vi "Vision_Processing_R_R10.vi"(0 "Current State":T2(ring), 1 "Image Dst":T6=refnum, 2 "Inpute Image":T6=refnum, 3 "Startup Flag":bool, 5 "Current ROI Descriptor":T11={"Global Rectangle"=[0, 0, 640, 480], "Contours"=[{"ID"=enum."External", "Type"=12, "Coordinates"=[0, 0, 640, 480, 0]}]} {"Contours"."Type" items=["No Selection", "Point", "Line", "Rectangle", "Oval", "Polygon", "Freehand Region", "Annulus", "Unused2", "Unused3", "Broken Line", "Freehand Line", "Rotated Rectangle"]}, 6 "Avg Score - Last":dbl=923.3457641601562, 7 "error in (no error)":errorcluster, 8 "Current Settings":T9={"Curve Parameters"={"Extraction Mode"=1, "Edge Threshold"=150, "Edge Filter Size"=0, "Min Length"=15, "Row Search Step Size"=10, "Col Search Step Size"=10, "Max Endpoint Gap"=2, "Closed"=TRUE, "Subpixel"=TRUE}, "Match Mode"={"Rotation"=TRUE, "Scale"=TRUE, "Occlusion"=FALSE, "Reserved"=FALSE, "Reserved"=FALSE, "Reserved"=FALSE}, "Range Settings"=[{"Match Constraints"=0, "Min"=-5.0, "Max"=5.0}, {"Match Constraints"=1, "Min"=20.0, "Max"=170.0}, {"Match Constraints"=2, "Min"=0.0, "Max"=20.0}], "Number of Matches"=1, "Minimum Match Score"=800.0, "SubPixel Accuracy"=TRUE, "Adv. Geometric Match Options 2"=[{"Setup Data Item"=20, "Item Value"=0.0}, {"Setup Data Item"=22, "Item Value"=1.0}]} {"Curve Parameters"."Extraction Mode" items=["Normal", "Uniform Regions"]; "Curve Parameters"."Edge Filter Size" items=["Fine", "Normal", "Contour Tracing"]; "Curve Parameters"."Max Endpoint Gap" min=0; "Curve Parameters"."Col Search Step Size" min=1 max=255 step=1; "Curve Parameters"."Row Search Step Size" min=1 max=255 step=1; "Curve Parameters"."Min Length" min=0; "Curve Parameters"."Edge Threshold" min=1 max=350 step=1; "Range Settings"."Max" format="%.2f"; "Range Settings"."Min" format="%.2f"; "Range Settings"."Match Constraints" items=["Rotation Angle (degrees)", "Scale Factor (%)", "Occlusion (%)"]; "Adv. Geometric Match Options 2"."Setup Data Item" items=["Curve Extraction Mode", "Curve Edge Threshold", "Curve Edge Filter Size", "Min Curve Length", "Curve Row Search Step Size", "Curve Col Search Step Size", "Curve Max Endpoint Gap", "Extract Closed Curves", "Enable Subpixel Curve Extraction", "Enable Correlation Score", "Enable Subpixel Accuracy", "Subpixel Iterations", "Subpixel Tolerance", "Initial Match List Length", "Enable Target Template Curve Score", "Min Match Separation Distance", "Min Match Separation Angle", "Min Match Separation Scale", "Max Match Overlap", "Enable Coarse Result", "Enable Calibration Support", "Enable Contrast Reversal", "Search Strategy", "Refinement Match Factor", "Subpixel Match Factor"]}, 9 "Sub Beacon Search Enable":bool[](array[boolean])=[FALSE, FALSE, FALSE, FALSE, FALSE], 10 "History Data - IN":T5={"Valid Beacon History - in"=[FALSE, FALSE, TRUE, FALSE, FALSE, FALSE, FALSE, FALSE, FALSE, FALSE, FALSE, FALSE, FALSE, FALSE, FALSE, TRUE, FALSE, FALSE, FALSE, FALSE], "Valid Score History"=[0.0, 0.0, 934.5453491210938, 891.6079711914062, 0.0, 0.0, 0.0, 0.0, 0.0, 0.0, 0.0, 0.0, 884.2328491210938, 0.0, 0.0, 902.6854858398438, 0.0, 0.0, 0.0, 0.0], "Valid Scale History"=[0.0, 0.0, 51.11858367919922, 10.0, 0.0, 0.0, 0.0, 0.0, 0.0, 0.0, 0.0, 0.0, 10.0, 0.0, 0.0, 55.87311935424805, 0.0, 0.0, 0.0, 0.0]} {"Valid Scale History" format="%#_13g"; "Valid Score History" format="%#_13g"}, 13 "Avg Scale - Last":dbl=54.029449462890625, 16 "History Size":i32=20) -> (11 "Avg Scale":dbl=54.029449462890625, 12 "Avg Score":dbl=923.3457641601562, 14 "Tracking Info 1":T1={"Tracking Coordinates"={"X"=0.0, "Y"=0.0}, "Current Valid"=FALSE, "Current State - Out"=enum."Sub - 2", "Setting Values"={"Min Scale"=17.429317474365234, "Max Scale"=90.62958145141602, "Min Score"=850.0}}, 15 "Next Main ROI Descriptor":T3={"Global Rectangle"=[0, 0, 640, 480], "Contours"=[{"ID"=enum."External", "Type"=12, "Coordinates"=[0, 0, 640, 480, 0]}]} {"Contours"."Type" items=["No Selection", "Point", "Line", "Rectangle", "Oval", "Polygon", "Freehand Region", "Annulus", "Unused2", "Unused3", "Broken Line", "Freehand Line", "Rotated Rectangle"]}, 17 "Beacon - Scales":sgl[](array[numeric]), 18 "History Data - Out":T4={"Valid Beacon History\nOut"=[FALSE, FALSE, TRUE, FALSE, FALSE, FALSE, FALSE, FALSE, FALSE, FALSE, FALSE, FALSE, FALSE, FALSE, FALSE, TRUE, FALSE, FALSE, FALSE, FALSE], "Valid Score History\nOut"=[0.0, 0.0, 934.5453491210938, 891.6079711914062, 0.0, 0.0, 0.0, 0.0, 0.0, 0.0, 0.0, 0.0, 884.2328491210938, 0.0, 0.0, 902.6854858398438, 0.0, 0.0, 0.0, 0.0], "Valid Scale History\nOut"=[0.0, 0.0, 51.11858367919922, 10.0, 0.0, 0.0, 0.0, 0.0, 0.0, 0.0, 0.0, 0.0, 10.0, 0.0, 0.0, 55.87311935424805, 0.0, 0.0, 0.0, 0.0]} {"Valid Scale History\nOut" format="%#_13g"; "Valid Score History\nOut" format="%#_13g"}, 19 "Y Coordinates":sgl[](array[numeric]), 20 "Beacons Found":bool[](array[boolean]), 21 "X Coordinates":sgl[](array[numeric]), 22 "Next State":T2(ring), 23 "Lock Status":bool, 24 "Startup Flag - out":bool, 25 "New Settings":T9={"Curve Parameters"={"Extraction Mode"=1, "Edge Threshold"=150, "Edge Filter Size"=0, "Min Length"=15, "Row Search Step Size"=10, "Col Search Step Size"=10, "Max Endpoint Gap"=2, "Closed"=TRUE, "Subpixel"=TRUE}, "Match Mode"={"Rotation"=TRUE, "Scale"=TRUE, "Occlusion"=FALSE, "Reserved"=FALSE, "Reserved"=FALSE, "Reserved"=FALSE}, "Range Settings"=[{"Match Constraints"=0, "Min"=-5.0, "Max"=5.0}, {"Match Constraints"=1, "Min"=20.0, "Max"=170.0}, {"Match Constraints"=2, "Min"=0.0, "Max"=20.0}], "Number of Matches"=1, "Minimum Match Score"=800.0, "SubPixel Accuracy"=TRUE, "Adv. Geometric Match Options 2"=[{"Setup Data Item"=20, "Item Value"=0.0}, {"Setup Data Item"=22, "Item Value"=1.0}]} {"Curve Parameters"."Extraction Mode" items=["Normal", "Uniform Regions"]; "Curve Parameters"."Edge Filter Size" items=["Fine", "Normal", "Contour Tracing"]; "Curve Parameters"."Max Endpoint Gap" min=0; "Curve Parameters"."Col Search Step Size" min=1 max=255 step=1; "Curve Parameters"."Row Search Step Size" min=1 max=255 step=1; "Curve Parameters"."Min Length" min=0; "Curve Parameters"."Edge Threshold" min=1 max=350 step=1; "Range Settings"."Max" format="%.2f"; "Range Settings"."Min" format="%.2f"; "Range Settings"."Match Constraints" items=["Rotation Angle (degrees)", "Scale Factor (%)", "Occlusion (%)"]}, 27 "Right Image 2":T6(plugin-control))   [LabVIEW 2015]
uses:
  <vilib>/vision/Image Controls.llb/IMAQ Image.ctl
  <vilib>/vision/Pattern Matching.llb/IMAQ Curve Parameters.ctl
  <vilib>/vision/Pattern Matching.llb/IMAQ Match Range Setting.ctl
panel:
  in  "ROBOT STATE(fwd, bwd, neither)":i32
  out "beacon - Scores":sgl[](array[numeric])
  in  "Minimum Score\nNormal 5":dbl=750.0
  in  "Minimum Score\nSub 4":dbl=850.0
  in  "Minimum Score\nSub 3":dbl=900.0
  in  "Minimum Score\nSub 2":dbl=950.0
  in  "Sub - 4 - FIle Path":path=path "/home/lvuser/natinst/bin/BeaconTemplates/4_beacons_right.png"
  in  "3 / 2\nTransition Scale":sgl=100.0
  in  "Score\nCushion- tight":dbl=75.0
  in  "Main ROI Decay\nper Fail (Vertical)":i32=5
  in  "ROI_factor(Horiztonal) (2 b)":sgl=2.0
  in  "ROI_factor(vertical) (2 b)":sgl=2.5
  in  "Sub - 2 File Path":path=path "/home/lvuser/natinst/bin/BeaconTemplates/2_beacons_right.png"
  out "Scale Decay \nFactor":dbl=18.300065994262695
  in  "ScoreDecay \nFactor":dbl=5.0
  in  "Valid Treshold\nfor Lock":i16=3
  in  "Horiztonall Beacon \nCushion (pixels)":sgl=20.0
  out "New Min Score":dbl=800.0
  out "New Low Scale":dbl=20.0
  out "New high Scale":dbl=170.0
  in  "Absolute\nMinimum Score":dbl=750.0
  in  "Absolute\nMaximum Scale":dbl=300.0
  in  "Absolute\nMinimum Scale":dbl=10.0
  in  "Default No Lock\nSetting Values":T10={"Min Scale"=20.0, "Max Scale"=170.0, "Min Score"=800.0}
  in  "Score\nCushion":dbl=100.0
  out "Scale \nCushion":dbl=18.300065994262695
  in  "5 / 2\nTransition Scale":sgl=60.0
  in  "4 / 2\nTransition Scale":sgl=85.0
  in  "Timeout \nThrehsold":i32=1000
  in  "Main ROI Decay\nper Fail (Horiztonal)":i32=25
  in  "ROI_factor(Horiztonal) (4 b)":sgl=5.0
  in  "ROI_factor(vertical) (4 b)":sgl=1.5
  in  "ROI_factor(vertical) (5 b)":sgl=2.7
  in  "ROI_factor(Horiztonal) (5 b)":sgl=4.7
  out "Current  Score":sgl=908.09845
  out "Current  Scale":sgl=51.91207
  in  "Fail Count - In":i32
  in  "Sub Beacon Template File Path - ARRAY":path[](array[path])=[path "/home/lvuser/natinst/bin/BeaconTemplates/Sub1.png", path "/home/lvuser/natinst/bin/BeaconTemplates/Sub2.png", path "/home/lvuser/natinst/bin/BeaconTemplates/Sub3.png", path "/home/lvuser/natinst/bin/BeaconTemplates/Sub4.png", path "/home/lvuser/natinst/bin/BeaconTemplates/Sub5.png"]
  in  "Sub - 3 - FIle Path":path=path "/home/lvuser/natinst/bin/BeaconTemplates/3_beacons_right.png"
  in  "Normal - 5 - File Path":path=path "/home/lvuser/natinst/bin/BeaconTemplates/5_beacons.png"
  # "INPUTS"
  # "FILE PATHS"
  # "CONFIG"
  # "OUTPUTS"
  # "************"
  # "Range"
  # "Range"
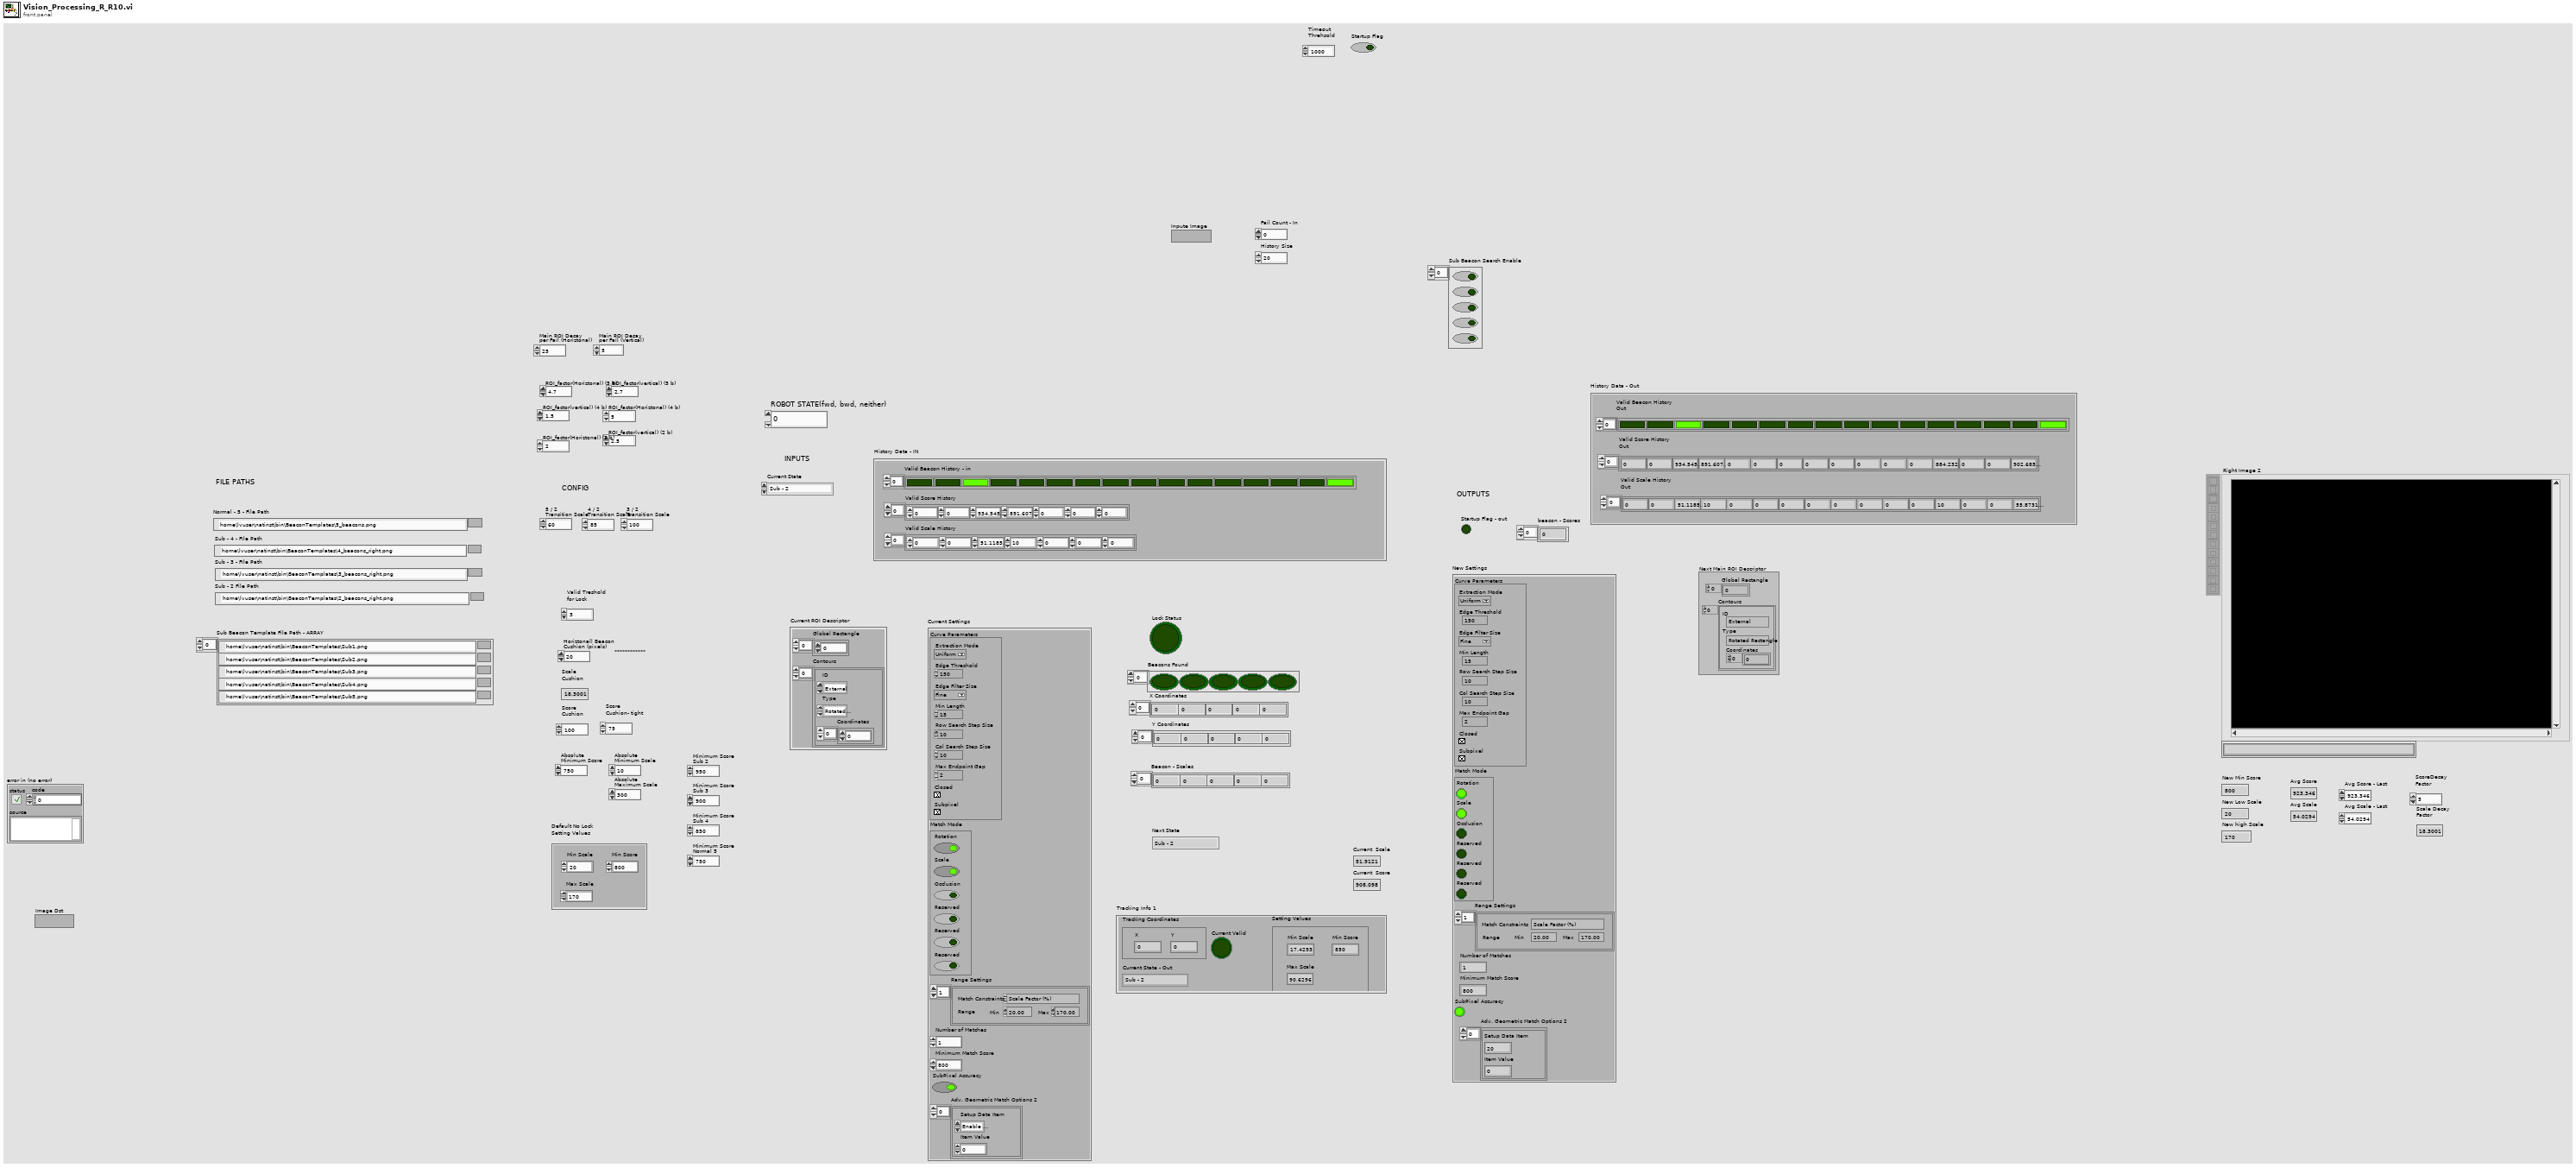
[diagram p1: front panel]
types:
  T1 = cluster{"Tracking Coordinates":cluster{"X":dbl, "Y":dbl}, "Current Valid":bool, "Current State - Out":enum16{"Sub - 2", "Sub - 3", "Sub - 4", "Normal - 5"}, "Setting Values":cluster{"Min Scale":dbl, "Max Scale":dbl, "Min Score":dbl}}
  T2 = enum16{"Sub - 2", "Sub - 3", "Sub - 4", "Normal - 5"}
  T3 = typedef "ROI Descriptor" = cluster{"Global Rectangle":i32[], "Contours":cluster{"ID":enum32{"External", "Internal"}, "Type":u32, "Coordinates":i32[]}[]}
  T4 = cluster{"Valid Beacon History\nOut":bool[], "Valid Score History\nOut":dbl[], "Valid Scale History\nOut":dbl[]}
  T5 = cluster{"Valid Beacon History - in":bool[], "Valid Score History":dbl[], "Valid Scale History":dbl[]}
  T6 = typedef "IMAQ Image.ctl" = refnum<image>
  T7 = typedef "IMAQ Curve Parameters.ctl" = cluster{"Extraction Mode":u32, "Edge Threshold":i32, "Edge Filter Size":u32, "Min Length":i32, "Row Search Step Size":i32, "Col Search Step Size":i32, "Max Endpoint Gap":i32, "Closed":bool, "Subpixel":bool}
  T8 = typedef "IMAQ Match Range Setting.ctl" = cluster{"Match Constraints":u32, "Min":dbl, "Max":dbl}
  T9 = cluster{"Curve Parameters":T7, "Match Mode":cluster{"Rotation":bool, "Scale":bool, "Occlusion":bool, "Reserved":bool, "Reserved":bool, "Reserved":bool}, "Range Settings":T8[], "Number of Matches":i32, "Minimum Match Score":sgl, "SubPixel Accuracy":bool, "Adv. Geometric Match Options 2":cluster{"Setup Data Item":u16, "Item Value":dbl}[]}
  T10 = cluster{"Min Scale":dbl, "Max Scale":dbl, "Min Score":dbl}
  T11 = cluster{"Global Rectangle":i32[], "Contours":cluster{"ID":enum32{"External", "Internal"}, "Type":u32, "Coordinates":i32[]}[]}
  T12 = typedef "IMAQ GM Match Report.ctl" = cluster{"Position":cluster{"x":sgl, "y":sgl}, "Angle":sgl, "Scale":sgl, "Score":sgl, "Bounding Box":cluster{"x":sgl, "y":sgl}[], "Contrast Reversed":bool, "Occlusion %":sgl, "Template Target Curve Score":sgl, "Target Template Curve Score":sgl, "Correlation Score":sgl}
  T13 = cluster{"Matches (Geometric Matching 1)[0]":T12, "Matches (Geometric Matching 1)[1]":T12, "Matches (Geometric Matching 1)[2]":T12, "Matches (Geometric Matching 1)[3]":T12, "Matches (Geometric Matching 1)[4]":T12, "Matches (Geometric Matching 1)[5]":T12, "Matches (Geometric Matching 1)[6]":T12, "Matches (Geometric Matching 1)[7]":T12, "Matches (Geometric Matching 1)[8]":T12}
  T14 = cluster{"Bounding Box[0]":cluster{"x":sgl, "y":sgl}, "Bounding Box[1]":cluster{"x":sgl, "y":sgl}, "Bounding Box[2]":cluster{"x":sgl, "y":sgl}, "Bounding Box[3]":cluster{"x":sgl, "y":sgl}, "Bounding Box[4]":cluster{"x":sgl, "y":sgl}, "Bounding Box[5]":cluster{"x":sgl, "y":sgl}, "Bounding Box[6]":cluster{"x":sgl, "y":sgl}, "Bounding Box[7]":cluster{"x":sgl, "y":sgl}, "Bounding Box[8]":cluster{"x":sgl, "y":sgl}}
  T15 = cluster{"index":u32, "Absolute\nMinimum Scale":dbl, "Absolute\nMaximum Scale":dbl}
  T16 = cluster{"New Low Scale":dbl, "New high Scale":dbl, "New Min Score":dbl}
  T17 = cluster{"Position":cluster{"x":sgl, "y":sgl}, bool, "Current State - Out":enum16{"Sub - 2", "Sub - 3", "Sub - 4", "Normal - 5"}, cluster{"New Low Scale":dbl, "New high Scale":dbl, "New Min Score":dbl}}
  T18 = cluster{"Position":cluster{"x":sgl, "y":sgl}, bool, "Current State":enum16{"Sub - 2", "Sub - 3", "Sub - 4", "Normal - 5"}, cluster{"New Low Scale":dbl, "New high Scale":dbl, "New Min Score":dbl}}
  T19 = typedef "IMAQ Rectangle" = cluster{"Left":i32, "Top":i32, "Right":i32, "Bottom":i32, "Rotation":dbl}
  T20 = cluster{"index":u32, "Min Scale":dbl, "Max Scale":dbl}
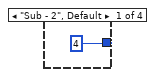
[diagram p3: hidden frame]
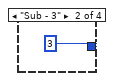
[diagram p4: hidden frame]
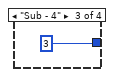
[diagram p5: hidden frame]
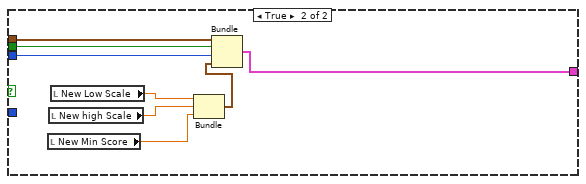
[diagram p6: hidden frame]
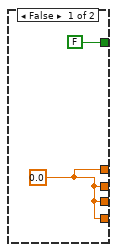
[diagram p7: hidden frame]
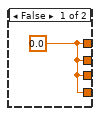
[diagram p8: hidden frame]
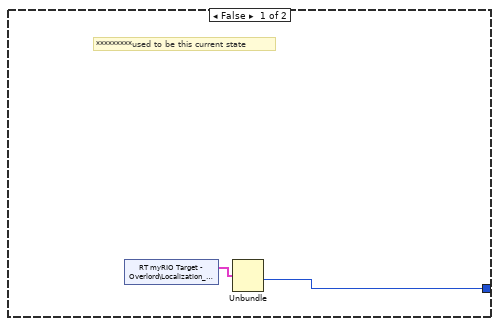
[diagram p12: hidden frame]
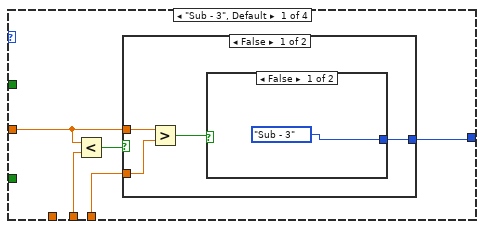
[diagram p13: hidden frame]
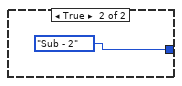
[diagram p14: hidden frame]
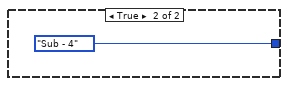
[diagram p15: hidden frame]
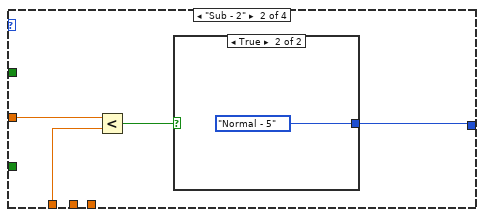
[diagram p16: hidden frame]
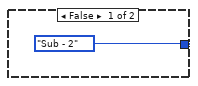
[diagram p17: hidden frame]
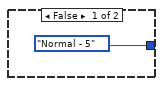
[diagram p18: hidden frame]
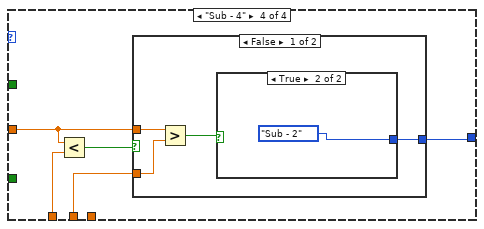
[diagram p19: hidden frame]
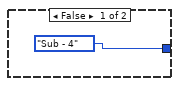
[diagram p20: hidden frame]
diagram:
  (unwired) enum16{"Short Range", "Long Range"}."Short Range"
  # "Next Settings"
  n1 = flat-sequence {
    tunnel: [w8] -> w3
    tunnel: [w7] -> w2
    tunnel: ["Image Dst"] -> w1
    tunnel: w3 -> [w160]
    tunnel: w2 -> [w158]
    tunnel: w1 -> [w159]
    frame #0 {
      # "APPLY FILTERING"
      n2 = call "Camera - Filtering"("Image In"="Inpute Image", "Image Dst"="Image Dst", "error in"="error in (no error)") -> ("Image Out"=w8:T6, "error out"=w7:errorcluster)  [unwired: 23 in]
    }
    frame #1 {
      w41 = u32 1 ("index")
      w122 = u32 1 ("index")
      w143 = u8 5
      # "*************************************************************************************************"
      # "Current Scale"
      # "Lower Scale"
      # "Upper Scale"
      # "Scale"
      # "Start up Template"
      # "Image Lock"
      # "Update Tracking Coordinates"
      # "CURRENT VALID"
      # "*************"
      # "Beacon - Y"
      # "Beacon - X"
      # "Beacons Found"
      # "Build ROI for Individual Beacons Based on Main Bounding Box"
      # "Starting X Lower Bound"
      # "Length of\nIndividual Beacon ROI"
      # "Length of Bounding Box"
      # "Choose ROI Factor based on Next State"
      # "Current Match"
      # "Current ROI"
      # "Image Lock"
      # "Force SR on Startup"
      # "Valid History"
      # "Draw ROI and stuff on outputi mage"
      # "Pull Down Startup IF Already True and Lock\nOtherwise don't update"
      # "Next Settings"
      # "Apply Limits to Settings"
      # "Scale"
      # "Min Score"
      # "Lower Scale"
      # "Upper Scale"
      # "Current Settings"
      # "Current Min\n& Max Scale"
      # "Current Valid"
      # "Update Search Settings"
      # "Update Template State"
      # "Calculate Average Scale/Score"
      # "max avg"
      # "Min Required to use avarage"
      # "Valid  Ccount\n(up to 3)"
      # "****# of previous in history that must be true\nin order for position to be considered \"locked\""
      # "Update Shift Arrays"
      # "# of Beacons Found to be valid"
      # "# of beacons"
      # "Matches"
      # "image out"
      n3 = Select(t=T2."Sub - 2", s="Startup Flag", f="Current State") -> (s? t:f=w50:T2)
      n4 = case shown="\"Sub - 2\"" w50 {
        tunnel: w160 -> [w540 w572 w603 w638]
        tunnel: w159 -> [w539 w571 w602 w637]
        tunnel: "Current ROI Descriptor" -> [w538 w570 w600 w636]
        tunnel: "Current Settings" -> [w537 w569 w599 w635]
        tunnel: [w533 w565 w596 w631] -> w86
        tunnel: [w532 w564 w597 w630] -> w106
        tunnel: [w530 w562 w598 w628] -> w151
        tunnel: w158 -> [_ _ w601 w627]
        tunnel: "Sub Beacon Search Enable" -> [w531 w563 w604 w626]
        tunnel: [sgl 3.0 ("y") sgl 2.0 ("y") 4.0 sgl 5.0 ("y")] -> w156
        tunnel: [w528 w560 w594 w624] -> w155
        tunnel: [2 1 3 4] -> w152
        frame "Sub - 3" {
          n5 = call "Short Range 2"("Image In"=w540, "Image Dst"=w539, "ROI Descriptor (Geometric Matching 1)"=w538, "Settings (Geometric Matching 1)"=w537, "Template File Path (Geometric Matching 1)"="Sub - 3 - FIle Path") -> ("Image Out"=w532:T6, "Matches (Geometric Matching 1)"=w533:T12[], "Number of Matches (Geometric Matching 1)"=w534:i32, "error out"=w528:errorcluster)  [unwired: 19 in]
          n6 = Equal?(x=w534, y=1) -> (x = y?=w535:bool)
          n7 = case shown="True" w535 {
            tunnel: w531 -> [w548 w551]
            tunnel: [w541 w552] -> w530
            frame False {
              w542 = FALSE
              # "F"
              # "No Main Found,\nDon't Search any Subs"
              n8 = Replace Array Subset(array=w548, new element #1=w542, index #1=0 ("y"), new element #2=w542, index #2=1 ("y"), new element #3=w542, index #3=2 ("y"), new element #4=w542, index #4=3 ("y"), new element #5=w542, index #5=4 ("y")) -> (w541:bool[])
            }
            frame True {
              w550 = TRUE
              w549 = FALSE
              n9 = Replace Array Subset(array=w551, new element #1=w549, index #1=0 ("y"), new element #2=w549, index #2=1 ("y"), new element #3=w550, index #3=2 ("y"), new element #4=w550, index #4=3 ("y"), new element #5=w550, index #5=4 ("y")) -> (w552:bool[])
            }
          }
        }
        frame "Sub - 2" {
          n10 = call "Short Range"("Image In"=w572, "Image Dst"=w571, "ROI Descriptor (Geometric Matching 1)"=w570, "Settings (Geometric Matching 1)"=w569, "Template File Path (Geometric Matching 1)"="Sub - 2 File Path") -> ("Image Out"=w564:T6, "Matches (Geometric Matching 1)"=w565:T12[], "Number of Matches (Geometric Matching 1)"=w566:i32, "error out"=w560:errorcluster)  [unwired: 19 in]
          n11 = Equal?(x=w566, y=1) -> (x = y?=w567:bool)
          n12 = case shown="True" w567 {
            tunnel: w563 -> [w580 w583]
            tunnel: [w573 w584] -> w562
            frame False {
              w574 = FALSE
              # "F"
              # "No Main Found,\nDon't Search any Subs"
              n13 = Replace Array Subset(array=w580, new element #1=w574, index #1=0 ("y"), new element #2=w574, index #2=1 ("y"), new element #3=w574, index #3=2 ("y"), new element #4=w574, index #4=3 ("y"), new element #5=w574, index #5=4 ("y")) -> (w573:bool[])
            }
            frame True {
              w582 = TRUE
              w581 = FALSE
              # "Search for specific Beacons"
              n14 = Replace Array Subset(array=w583, new element #1=w581, index #1=0 ("y"), new element #2=w581, index #2=1 ("y"), new element #3=w581, index #3=2 ("y"), new element #4=w582, index #4=3 ("y"), new element #5=w582, index #5=4 ("y")) -> (w584:bool[])
            }
          }
        }
        frame "Sub - 4" {
          # "**Make sure this selects the \nappropriate beacons to search for!!"
          n15 = call "Dumping Range"("Image In"=w603, "Image Dst"=w602, "ROI Descriptor (Geometric Matching 1)"=w600, "Settings (Geometric Matching 1)"=w599, "Template File Path (Geometric Matching 1)"="Sub - 4 - FIle Path", "error in"=w601) -> ("Image Out"=w597:T6, "Matches (Geometric Matching 1)"=w596:T12[], "Number of Matches (Geometric Matching 1)"=w593:i32, "error out"=w594:errorcluster)  [unwired: 18 in]
          n16 = Equal?(x=w593, y=1) -> (x = y?=w591:bool)
          n17 = case shown="True" w591 {
            tunnel: w604 -> [w613 w616]
            tunnel: [w606 w617] -> w598
            frame False {
              w607 = FALSE
              # "F"
              # "No Main Found,\nDon't Search any Subs"
              n18 = Replace Array Subset(array=w613, new element #1=w607, index #1=0 ("y"), new element #2=w607, index #2=1 ("y"), new element #3=w607, index #3=2 ("y"), new element #4=w607, index #4=3 ("y"), new element #5=w607, index #5=4 ("y")) -> (w606:bool[])
            }
            frame True {
              w615 = TRUE
              n19 = Replace Array Subset(array=w616, new element #1=FALSE, index #1=0 ("y"), new element #2=w615, index #2=1 ("y"), new element #3=w615, index #3=2 ("y"), new element #4=w615, index #4=3 ("y"), new element #5=w615, index #5=4 ("y")) -> (w617:bool[])
            }
          }
        }
        frame "Normal - 5" {
          n20 = call "Long Range"("Image In"=w638, "Image Dst"=w637, "ROI Descriptor (Geometric Matching 1)"=w636, "Settings (Geometric Matching 1)"=w635, "Template File Path (Geometric Matching 1)"="Normal - 5 - File Path", "error in"=w627) -> ("Image Out"=w630:T6, "Matches (Geometric Matching 1)"=w631:T12[], "Number of Matches (Geometric Matching 1)"=w633:i32, "error out"=w624:errorcluster)  [unwired: 18 in]
          n21 = Equal?(x=w633, y=1) -> (x = y?=w629:bool)
          n22 = case shown="True" w629 {
            tunnel: w626 -> [w646 w648]
            tunnel: [w639 w647] -> w628
            frame False {
              w640 = FALSE
              # "F"
              # "No Main Found,\nDon't Search any Subs"
              n23 = Replace Array Subset(array=w646, new element #1=w640, index #1=0 ("y"), new element #2=w640, index #2=1 ("y"), new element #3=w640, index #3=2 ("y"), new element #4=w640, index #4=3 ("y"), new element #5=w640, index #5=4 ("y")) -> (w639:bool[])
            }
            frame True {
              w649 = TRUE
              # "T"
              # "Search for ALL Beacons"
              n24 = Replace Array Subset(array=w648, new element #1=w649, index #1=0 ("y"), new element #2=w649, index #2=1 ("y"), new element #3=w649, index #3=2 ("y"), new element #4=w649, index #4=3 ("y"), new element #5=w649, index #5=4 ("y")) -> (w647:bool[])
            }
          }
        }
      }
      n25 = Array To Cluster(array=w86) -> (cluster=w76:T13)
      n26 = Unbundle By Name(w76) -> ("Matches (Geometric Matching 1)[0].Position"=w52:cluster{"x":sgl, "y":sgl}, "Matches (Geometric Matching 1)[0].Bounding Box"=w74:cluster{"x":sgl, "y":sgl}[], "Matches (Geometric Matching 1)[0].Scale"=w31:sgl, "Matches (Geometric Matching 1)[0].Score"=w113:sgl)
      "Current  Scale" <- w31
      "Current  Score" <- w113
      n27 = Array To Cluster(array=w74) -> (cluster=w75:T14)
      n28 = Unbundle By Name(w75) -> ("Bounding Box[0].x"=w65:sgl, "Bounding Box[0].y"=w64:sgl, "Bounding Box[2].x"=w63:sgl, "Bounding Box[2].y"=w62:sgl)
      n29 = Bundle("x"=w65, "y"=w64, "x"=w63, "y"=w62) -> (w60:cluster{"x":sgl, "y":sgl, "x":sgl, "y":sgl})  [unwired: 1 in]
      n30 = call "IMAQ Overlay Rectangle"("Rectangle"=w60, "Image"=w106) -> ("Image Out"=w61:T6)  [unwired: 8 in, 1 out]
      n31 = Subtract(x=w63, y=w65) -> (x-y=w69:sgl)
      n32 = Divide(x=w69, y=w156) -> (x/y=w71:dbl)
      n33 = Multiply(x="Horiztonall Beacon \nCushion (pixels)", y=w31) -> (x*y=w59:sgl)
      n34 = Divide(x=w59, y=sgl 100.0) -> (x/y=w56:sgl)
      n35 = Subtract(x=w64, y=w56) -> (x-y=w72:sgl)
      n36 = Add(x=w56, y=w62) -> (x+y=w73:sgl)
      n37 = for {
        N: 5 -> [_]
        tunnel: w151 -> [w251] mode=indexing
        shift-right: [w245] -> _
        shift-left: w65 -> [w250]
        tunnel: w71 -> [w249]
        tunnel: w72 -> [w242]
        tunnel: w73 -> [w241]
        tunnel: [w248] -> w67 mode=indexing
        tunnel: w56 -> [w243]
        # "Divide Bounding Box"
        # "Upper Bound of Current is\nLower Bound for Next"
        n38 = case shown="True" w251 {
          tunnel: w250 -> [w252 w253]
          tunnel: w249 -> [_ w255]
          tunnel: [w252 w254] -> w245
          tunnel: [w252 w253] -> w247
          frame False {
            # "Don't Care"
          }
          frame True {
            # "X Lower Bound"
            n39 = Add(x=w253, y=w255) -> (x+y=w254:dbl)
          }
        }
        n40 = Subtract(x=w247, y=w243) -> (x-y=w246:dbl)
        n41 = Add(x=w245, y=w243) -> (x+y=w244:dbl)
        n42 = call "Bound_RO_R_R0I.vi"("Bottom Right - Y"=w241, "Right - X"=w244, "Top Left - Y"=w242, "Top  Left - x"=w246) -> ("ROI Descriptor"=w248:T3)  [unwired: 7 in]
      }
      n43 = local read "Absolute\nMaximum Scale"() -> (w32:dbl)
      n44 = local read "Absolute\nMinimum Scale"() -> (w33:dbl)
      n45 = local read "Scale \nCushion"() -> (w30:dbl)
      n46 = Add(x=w31, y=w30) -> (x+y=w28:dbl)
      n47 = Subtract(x=w31, y=w30) -> (x-y=w29:dbl)
      n48 = Less?(x=w29, y=w33) -> (x < y?=w37:bool)
      n49 = Greater?(x=w28, y=w32) -> (0:w34:bool)
      n50 = Greater?(x=w29, y=w28) -> (0:w38:bool)
      n51 = Less?(x=w28, y=w29) -> (x < y?=w35:bool)
      n52 = Or(x=w37, y=w38) -> (x .or. y?=w39:bool)
      n53 = Or(x=w34, y=w35) -> (x .or. y?=w36:bool)
      n54 = Select(t=w33, s=w39, f=w29) -> (s? t:f=w27:dbl)
      n55 = Select(t=w32, s=w36, f=w28) -> (s? t:f=w26:dbl)
      n56 = Unbundle By Name("Current Settings") -> ("Range Settings"=w22:T8[])
      n57 = Bundle("index"=w41, "Absolute\nMinimum Scale"=w27, "Absolute\nMaximum Scale"=w26) -> (w40:T15)  [unwired: 1 in]
      n58 = Replace Array Subset(array=w22, new element=w40, index=w41) -> (w25:T8[])
      n59 = Bundle By Name(cluster="Current Settings", "Range Settings"=w25) -> (w24:T9)
      n60 = for {
        N: 5 -> [_]
        tunnel: w106 -> [w218]
        tunnel: w155 -> [w217]
        tunnel: w67 -> [w210] mode=indexing
        tunnel: "Sub Beacon Template File Path - ARRAY" -> [w216] mode=indexing
        tunnel: [w215] -> w45 mode=indexing
        tunnel: [w214] -> w44 mode=indexing
        tunnel: [w213] -> w46 mode=indexing
        tunnel: w151 -> [w212] mode=indexing
        tunnel: w24 -> [w211]
        shift-right: [w208] -> w107
        shift-left: w61 -> [w209]
        tunnel: [w207] -> w97 mode=indexing
        tunnel: [w206] -> w16 mode=indexing
        n61 = case shown="True" w212 {
          tunnel: w218 -> [_ w233]
          tunnel: w217 -> [_ w232]
          tunnel: w210 -> [_ w231]
          tunnel: w216 -> [_ w230]
          tunnel: [w219 w226] -> w215
          tunnel: [w219 w225] -> w214
          tunnel: [FALSE w224] -> w213
          tunnel: w211 -> [_ w223]
          tunnel: [w219 w222] -> w207
          tunnel: [w219 w221] -> w206
          frame False {
            w219 = sgl 0.0 ("x")
          }
          frame True {
            n62 = call "Sub Beacon Pattern Match"("Image In"=w233, "ROI Descriptor (Geometric Matching 1)"=w231, "Settings (Geometric Matching 1)"=w223, "Template File Path (Geometric Matching 1)"=w230, "error in"=w232) -> ("Matches (Geometric Matching 1)"=w227:T12[], "Number of Matches (Geometric Matching 1)"=w228:i32)  [unwired: 19 in, 2 out]
            n63 = Equal?(x=w228, y=1) -> (x = y?=w224:bool)
            n64 = case shown="True" w224 {
              tunnel: w227 -> [_ w239]
              tunnel: [w234 w238] -> w226
              tunnel: [w234 w237] -> w225
              tunnel: [w234 w236] -> w222
              tunnel: [w234 w235] -> w221
              frame False {
                w234 = sgl 0.0 ("x")
              }
              frame True {
                n65 = Array To Cluster(array=w239) -> (cluster=w240:T13)
                n66 = Unbundle By Name(w240) -> ("Matches (Geometric Matching 1)[0].Position.x"=w238:sgl, "Matches (Geometric Matching 1)[0].Position.y"=w237:sgl, "Matches (Geometric Matching 1)[0].Scale"=w236:sgl, "Matches (Geometric Matching 1)[0].Score"=w235:sgl)
              }
            }
          }
        }
        n67 = call "IMAQ Overlay ROI"("ROI Descriptor"=w210, "Image"=w209) -> ("Image Out"=w208:T6)  [unwired: 8 in, 1 out]
      }
      "Beacons Found" <- w46
      "X Coordinates" <- w45
      "Y Coordinates" <- w44
      "Beacon - Scales" <- w97
      "beacon - Scores" <- w16
      n68 = Boolean To (0,1)(Boolean=w46) -> (0, 1=w153:i16[])
      n69 = Add Array Elements(numeric array=w153) -> (sum=w154:i16)
      n70 = Greater Or Equal?(x=w154, y=w152) -> (x >= y?=w51:bool)
      n71 = case shown="False" w51 {
        tunnel: "Fail Count - In" -> [w524 _]
        tunnel: [w523 u16 0] -> w136
        frame False {
          n72 = Increment(x=w524) -> (x+1=w523:i32)
        }
        frame True {
          # "reset fail count"
        }
      }
      n73 = Unbundle By Name("History Data - IN") -> ("Valid Beacon History - in"=w104:bool[], "Valid Score History"=w103:dbl[], "Valid Scale History"=w102:dbl[])
      n74 = Greater?(x=w136, y="Timeout \nThrehsold") -> (0:w53:bool)
      n75 = Decrement(x="History Size") -> (x-1=w149:i32)
      n76 = for {
        N: "History Size" -> [_]
        shift-right: [w501] -> w101
        shift-left: w104 -> [w489]
        tunnel: w149 -> [w497]
        shift-right: [w494] -> w100
        shift-left: w103 -> [w496]
        shift-right: [w493] -> w99
        shift-left: w102 -> [w495]
        tunnel: w113 -> [w492]
        tunnel: w31 -> [w491]
        tunnel: w51 -> [w490]
        i -> [w500]
        # "Reverse Index"
        n77 = Subtract(x=w497, y=w500) -> (x-y=w498:i32)
        n78 = Equal To 0?(x=w498) -> (x = 0?=w499:bool)
        n79 = case shown="True" w499 {
          tunnel: w498 -> [w502 w521]
          tunnel: w489 -> [w512 w514]
          tunnel: [w510 w513] -> w501
          tunnel: w490 -> [_ w522]
          tunnel: w496 -> [w507 w520]
          tunnel: w495 -> [w506 w519]
          tunnel: [w505 w517] -> w494
          tunnel: [w504 w518] -> w493
          tunnel: w492 -> [_ w516]
          tunnel: w491 -> [_ w515]
          frame False {
            # "Shift Old"
            n80 = Decrement(x=w502) -> (x-1=w503:i32)
            n81 = Index Array(array=w512, index=w503) -> (element=w511:bool)
            n82 = Index Array(array=w507, index=w503) -> (element=w509:dbl)
            n83 = Index Array(array=w506, index=w503) -> (element=w508:dbl)
            n84 = Replace Array Subset(array=w512, new element=w511, index=w502) -> (w510:bool[])
            n85 = Replace Array Subset(array=w507, new element=w509, index=w502) -> (w505:dbl[])
            n86 = Replace Array Subset(array=w506, new element=w508, index=w502) -> (w504:dbl[])
          }
          frame True {
            # "Scale"
            # "Score"
            # "Valid"
            # "insert New"
            n87 = Replace Array Subset(array=w520, new element=w516, index=w521) -> (w517:dbl[])
            n88 = Replace Array Subset(array=w519, new element=w515, index=w521) -> (w518:dbl[])
            n89 = Replace Array Subset(array=w514, new element=w522, index=w521) -> (w513:bool[])
          }
        }
      }
      n90 = Boolean To (0,1)(Boolean=w101) -> (0, 1=w147:i16[])
      n91 = Bundle("Valid Beacon History - in"=w101, "Valid Score History"=w100, "Valid Scale History"=w99) -> (→"History Data - Out":T5)  [unwired: 1 in]
      n92 = Add Array Elements(numeric array=w147) -> (sum=w148:i16)
      n93 = Greater Or Equal?(x=w148, y="Valid Treshold\nfor Lock") -> (x >= y?=w114:bool)
      "Lock Status" <- w114
      n94 = Initialize Array(u8 0, w143) -> (w145:u8[])
      n95 = while {
        shift-right: [w472] -> w141
        shift-left: w145 -> [w474]
        tunnel: w101 -> [w480] mode=indexing
        shift-right: [w478] -> w139
        shift-left: u8 0 -> [w481]
        tunnel: "History Size" -> [w479]
        tunnel: w143 -> [w471]
        i -> [w473]
        stop <- w475 stop-if-true
        # "Grab Last 2 Valid Indexes"
        n96 = case shown="True" w480 {
          tunnel: w481 -> [w483 w485]
          tunnel: [w483 w488] -> w478
          tunnel: w474 -> [w482 w487]
          tunnel: w473 -> [_ w486]
          tunnel: [w482 w484] -> w472
          frame False {
          }
          frame True {
            # "Update Index\nto use"
            # "Increment\nValid Count"
            n97 = Replace Array Subset(array=w487, new element=w486, index=w485) -> (w484:u8[])
            n98 = Increment(x=w485) -> (x+1=w488:u8)
          }
        }
        n99 = Greater?(x=w473, y=w479) -> (0:w476:bool)
        n100 = Greater Or Equal?(x=w478, y=w471) -> (x >= y?=w477:bool)
        n101 = Or(x=w477, y=w476) -> (x .or. y?=w475:bool)
      }
      n102 = Greater?(x=w139, y=u8 2) -> (0:w140:bool)
      n103 = case shown="True" w140 {
        tunnel: w139 -> [_ w455]
        tunnel: w141 -> [_ w461]
        tunnel: w100 -> [_ w460]
        tunnel: w99 -> [_ w459]
        tunnel: ["Avg Score - Last" w453] -> w111
        tunnel: ["Avg Scale - Last" w452] -> w9
        frame False {
        }
        frame True {
          w458 = 0.0
          n104 = for {
            N: w455 -> [_]
            tunnel: w461 -> [w468] mode=indexing
            tunnel: w460 -> [w470]
            tunnel: w459 -> [w469]
            shift-right: [w466] -> w457
            shift-left: w458 -> [w464]
            shift-right: [w467] -> w456
            shift-left: w458 -> [w463]
            # "Fetch Last Valid Values"
            n105 = Index Array(array=w470, index=w468) -> (element=w465:dbl)
            n106 = Index Array(array=w469, index=w468) -> (element=w462:dbl)
            n107 = Add(x=w465, y=w464) -> (x+y=w466:dbl)
            n108 = Add(x=w462, y=w463) -> (x+y=w467:dbl)
          }
          n109 = To Double Precision Float(number=w455) -> (double precision float=w454:dbl)
          n110 = Divide(x=w457, y=w454) -> (x/y=w453:dbl)
          n111 = Divide(x=w456, y=w454) -> (x/y=w452:dbl)
        }
      }
      "Avg Score" <- w111
      "Avg Scale" <- w9
      n112 = case shown="True" w114 {
        tunnel: w53 -> [_ w273]
        tunnel: "4 / 2\nTransition Scale" -> [_ w272]
        tunnel: "5 / 2\nTransition Scale" -> [_ w271]
        tunnel: w9 -> [_ w270]
        tunnel: w114 -> [_ w269]
        tunnel: [w265 w268] -> w42
        tunnel: "3 / 2\nTransition Scale" -> [_ w267]
        frame False {
          # "*********used to be this current state"
          n113 = shared-variable "RT myRIO Target - Overlord\\Localization_Variables_r0.lvlib\\Info - Left"() -> (w266:T1)  [unwired: 1 in, 1 out]
          n114 = Unbundle(w266) -> ("Current State - Out"=w265:T2)  [unwired: 3 out]
        }
        frame True {
          # "Timeout"
          n115 = local read "Current State"() -> (w274:T2)
          n116 = case shown="\"Normal - 5\"" w274 {
            tunnel: w269 -> [_ _ _ _]
            tunnel: w270 -> [w278 w290 w295 w301]
            tunnel: w273 -> [_ _ _ _]
            tunnel: w272 -> [w279 _ _ w300]
            tunnel: w271 -> [_ w287 w294 w303]
            tunnel: [w275 w288 w293 w299] -> w268
            tunnel: w267 -> [w276 _ _ _]
            frame "Sub - 3", Default {
              n117 = Less?(x=w278, y=w279) -> (x < y?=w277:bool)
              n118 = case shown="False" w277 {
                tunnel: w278 -> [w283 _]
                tunnel: [w280 T2."Sub - 4"] -> w275
                tunnel: w276 -> [w282 _]
                frame False {
                  n119 = Greater?(x=w283, y=w282) -> (0:w281:bool)
                  n120 = case shown="False" w281 {
                    tunnel: [T2."Sub - 3" T2."Sub - 2"] -> w280
                    frame False {
                    }
                    frame True {
                    }
                  }
                }
                frame True {
                }
              }
            }
            frame "Sub - 2" {
              n121 = Less?(x=w290, y=w287) -> (x < y?=w289:bool)
              n122 = case shown="True" w289 {
                tunnel: [T2."Sub - 2" T2."Normal - 5"] -> w288
                frame False {
                }
                frame True {
                }
              }
            }
            frame "Normal - 5" {
              # "If Out of Scale Range\nor Timeout"
              n123 = Greater?(x=w295, y=w294) -> (0:w296:bool)
              n124 = case shown="True" w296 {
                tunnel: [T2."Normal - 5" T2."Sub - 2"] -> w293
                frame False {
                }
                frame True {
                }
              }
            }
            frame "Sub - 4" {
              n125 = Less?(x=w301, y=w303) -> (x < y?=w302:bool)
              n126 = case shown="False" w302 {
                tunnel: w301 -> [w307 _]
                tunnel: [w304 T2."Normal - 5"] -> w299
                tunnel: w300 -> [w306 _]
                frame False {
                  n127 = Greater?(x=w307, y=w306) -> (0:w305:bool)
                  n128 = case shown="True" w305 {
                    tunnel: [T2."Sub - 4" T2."Sub - 2"] -> w304
                    frame False {
                    }
                    frame True {
                    }
                  }
                }
                frame True {
                }
              }
            }
          }
        }
      }
      "Next State" <- w42
      n129 = local read "Current State"() -> (w47:T2)
      n130 = Equal?(x=w47, y=w42) -> (x = y?=w43:bool)
      n131 = case shown="False" w43 {
        tunnel: w52 -> [w170 w205]
        tunnel: w51 -> [w167 w204]
        tunnel: w50 -> [_ w203]
        tunnel: [w166 w202] -> w15
        tunnel: w42 -> [w164 _]
        tunnel: w46 -> [w174 _]
        tunnel: w45 -> [w172 _]
        tunnel: w44 -> [w171 _]
        frame False {
          # "Beacon Index"
          # "Check if Tracking is Available for the Next Template State"
          n132 = case shown="\"Normal - 5\"" w164 {
            tunnel: [4 3 3 3] -> w169
            frame "Sub - 2", Default {
            }
            frame "Sub - 3" {
            }
            frame "Sub - 4" {
            }
            frame "Normal - 5" {
            }
          }
          n133 = Index Array(array=w174, index=w169) -> (element=w173:bool)
          n134 = case shown="True" w173 {
            tunnel: w172 -> [_ w193]
            tunnel: w171 -> [_ w192]
            tunnel: [w175 w189] -> w168
            tunnel: w170 -> [w175 w190]
            tunnel: w169 -> [_ w191]
            frame False {
            }
            frame True {
              w186 = sgl 0.4 ("y")
              n135 = Unbundle(w190) -> ("x"=w187:sgl, "y"=w185:sgl)
              n136 = Index Array(array=w193, index=w191) -> (element=w182:sgl)
              n137 = Index Array(array=w192, index=w191) -> (element=w183:sgl)
              n138 = Subtract(x=sgl 1.0, y=w186) -> (x-y=w184:sgl)
              n139 = Multiply(x=w184, y=w182) -> (x*y=w180:sgl)
              n140 = Multiply(x=w184, y=w183) -> (x*y=w178:sgl)
              n141 = Multiply(x=w186, y=w187) -> (x*y=w181:sgl)
              n142 = Multiply(x=w186, y=w185) -> (x*y=w179:sgl)
              n143 = Add(x=w181, y=w180) -> (x+y=w177:sgl)
              n144 = Add(x=w179, y=w178) -> (x+y=w176:sgl)
              n145 = Bundle(w177, w176) -> (w189:cluster{sgl, sgl})  [unwired: 1 in]
            }
          }
          n146 = local read "New Min Score"() -> (w161:dbl)
          n147 = local read "New high Scale"() -> (w162:dbl)
          n148 = local read "New Low Scale"() -> (w163:dbl)
          n149 = Bundle("New Low Scale"=w163, "New high Scale"=w162, "New Min Score"=w161) -> (w165:T16)  [unwired: 1 in]
          n150 = Bundle("Position"=w168, w167, "Current State - Out"=w164, w165) -> (w166:T17)  [unwired: 1 in]
        }
        frame True {
          n151 = local read "New Min Score"() -> (w199:dbl)
          n152 = local read "New high Scale"() -> (w200:dbl)
          n153 = local read "New Low Scale"() -> (w201:dbl)
          n154 = Bundle("New Low Scale"=w201, "New high Scale"=w200, "New Min Score"=w199) -> (w198:T16)  [unwired: 1 in]
          n155 = Bundle("Position"=w205, w204, "Current State"=w203, w198) -> (w202:T18)  [unwired: 1 in]
        }
      }
      "Tracking Info 1" <- w15
      n156 = Unbundle By Name("Current Settings") -> ("Minimum Match Score"=w133:sgl, "Range Settings"=w119:T8[])
      n157 = case shown="\"Normal - 5\"" w42 {
        tunnel: "ROI_factor(vertical) (5 b)" -> [_ _ w264]
        tunnel: "ROI_factor(Horiztonal) (5 b)" -> [_ _ w263]
        tunnel: "ROI_factor(vertical) (4 b)" -> [_ w261 _]
        tunnel: "ROI_factor(Horiztonal) (4 b)" -> [_ w260 _]
        tunnel: "ROI_factor(vertical) (2 b)" -> [w258 _ _]
        tunnel: "ROI_factor(Horiztonal) (2 b)" -> [w257 _ _]
        tunnel: [w258 w261 w264] -> w79
        tunnel: [w257 w260 w263] -> w78
        tunnel: "Minimum Score\nSub 2" -> [w256 _ _]
        tunnel: [w256 w259 w262] -> w18
        tunnel: "Minimum Score\nSub 3" -> [_ _ _]
        tunnel: "Minimum Score\nSub 4" -> [_ w259 _]
        tunnel: "Minimum Score\nNormal 5" -> [_ _ w262]
        frame "Sub - 2" {
        }
        frame "Sub - 4", Default {
        }
        frame "Normal - 5" {
        }
      }
      n158 = Index Array(array=w119, index=u32 1) -> (element=w132:T8)
      n159 = Unbundle(w132) -> ("Min"=w130:dbl, "Max"=w129:dbl)  [unwired: 1 out]
      n160 = And(x="Startup Flag", y=w114) -> (x .and. y?=w117:bool)
      n161 = case shown="True" w117 {
        tunnel: "Startup Flag" -> [w311 _]
        tunnel: [w311 FALSE] -> w116
        frame False {
        }
        frame True {
        }
      }
      "Startup Flag - out" <- w116
      n162 = call "Scaling and Mapping"("Signals"=w9) -> ("Scaled Signals"=w17:dynamicdata)  [unwired: 9 in, 1 out]
      n163 = To Single Precision Float(number=w17) -> (single precision float=w13:sgl)
      "Scale \nCushion" <- w13
      "Scale Decay \nFactor" <- w13
      n164 = call "Scaling and Mapping2"("Signals"=w9) -> ("Scaled Signals"=w11:dynamicdata)  [unwired: 9 in, 1 out]
      n165 = To Single Precision Float(number=w11) -> (single precision float=w10:sgl)
      n166 = case shown="True" w114 {
        tunnel: w51 -> [_ w371]
        tunnel: w111 -> [w325 w370]
        tunnel: w9 -> [w324 w369]
        tunnel: w133 -> [_ w368]
        tunnel: w130 -> [_ w367]
        tunnel: w129 -> [_ w366]
        tunnel: [w315 w345] -> w120
        tunnel: [w313 w357] -> w90
        tunnel: [w314 w356] -> w91
        tunnel: w13 -> [w327 w365]
        tunnel: "Score\nCushion" -> [w326 w364]
        tunnel: "ScoreDecay \nFactor" -> [_ w363]
        tunnel: w13 -> [_ w362]
        tunnel: "Current ROI Descriptor" -> [_ w358]
        tunnel: w86 -> [_ w359]
        tunnel: w79 -> [_ w361]
        tunnel: w78 -> [_ w360]
        tunnel: [w317 w355] -> w77
        tunnel: w43 -> [_ w350]
        tunnel: w42 -> [_ w349]
        tunnel: w18 -> [_ w346]
        tunnel: "ROBOT STATE(fwd, bwd, neither)" -> [_ w344]
        tunnel: w10 -> [_ w343]
        frame False {
          # "Check Lock Status of OTHER Cam,\n\nif True,\n\nthen use it's settings,\n\notherwise use default no lock"
          # "Initial ROI Descriptor"
          # "Apply No Lock Default for each Template"
          n167 = disable-structure shown="Disabled" {
            disable-tunnel: [w342 _] -> _
            disable-tunnel: [w341 _] -> _
            disable-tunnel: w327 -> [w340 _]
            disable-tunnel: w326 -> [w339 _]
            disable-tunnel: w325 -> [w338 _]
            disable-tunnel: w324 -> [w337 _]
            frame Disabled {
              n168 = Subtract(x=w338, y=w339) -> ()  [unwired: 1 out]
              n169 = Subtract(x=w337, y=w340) -> (x-y=w342:dbl)
              n170 = Add(x=w340, y=w337) -> (x+y=w341:dbl)
            }
            frame Enabled {
            }
          }
          n171 = shared-variable "RT myRIO Target - Overlord\\Localization_Variables_r0.lvlib\\Image Lock - L"() -> (w316:bool)  [unwired: 1 in, 1 out]
          n172 = case shown="True" w316 {
            tunnel: [w330 w334] -> w315
            tunnel: [w328 w333] -> w314
            tunnel: [w329 w332] -> w313
            frame False {
              n173 = Unbundle By Name("Default No Lock\nSetting Values") -> ("Min Score"=w330:dbl, "Min Scale"=w329:dbl, "Max Scale"=w328:dbl)
            }
            frame True {
              n174 = shared-variable "RT myRIO Target - Overlord\\Localization_Variables_r0.lvlib\\Info - Left"() -> (w336:T1)  [unwired: 1 in, 1 out]
              n175 = Unbundle(w336) -> ("Setting Values"=w335:T10)  [unwired: 3 out]
              n176 = Unbundle(w335) -> ("Min Scale"=w332:dbl, "Max Scale"=w333:dbl, "Min Score"=w334:dbl)
            }
          }
          n177 = Bundle(0, 0, 640, 480, 0) -> (w323:cluster{i32, i32, i32, i32, i32})  [unwired: 1 in]
          n178 = call "IMAQ Convert Rectangle to ROI"("Rectangle"=w323) -> ("ROI Descriptor"=w317:T3)  [unwired: 8 in, 1 out]
        }
        frame True {
          # "Score out"
          # "Apply Limits to ROI"
          n179 = case shown="False" w371 {
            tunnel: w370 -> [_ w421]
            tunnel: [w389 w418] -> w347
            tunnel: w369 -> [_ w420]
            tunnel: [w388 w400] -> w357
            tunnel: [w387 w399] -> w356
            tunnel: w367 -> [w394 _]
            tunnel: w366 -> [w393 _]
            tunnel: w368 -> [w392 _]
            tunnel: w365 -> [_ w402]
            tunnel: w364 -> [_ w419]
            tunnel: w363 -> [w391 _]
            tunnel: w362 -> [w390 _]
            tunnel: w361 -> [_ w409]
            tunnel: w360 -> [_ w408]
            tunnel: w359 -> [_ w407]
            tunnel: [w380 w398] -> w354
            tunnel: [w379 w406] -> w353
            tunnel: [w378 w397] -> w352
            tunnel: [w377 w405] -> w351
            tunnel: w358 -> [w385 _]
            tunnel: w350 -> [_ _]
            tunnel: w349 -> [_ w404]
            tunnel: w344 -> [_ w395]
            tunnel: w343 -> [w373 _]
            frame False {
              # "Decrement Score by"
              n180 = Subtract(x=w394, y=w390) -> (x-y=w388:dbl)
              n181 = Add(x=w390, y=w393) -> (x+y=w387:dbl)
              n182 = Subtract(x=w392, y=w391) -> (x-y=w389:dbl)
              n183 = call "IMAQ Convert ROI to Rectangle"("ROI Descriptor"=w385) -> ("Rectangle"=w386:T19)  [unwired: 8 in, 1 out]
              n184 = Unbundle By Name(w386) -> ("Left"=w384:i32, "Top"=w383:i32, "Right"=w382:i32, "Bottom"=w381:i32)
              n185 = Divide(x=w373, y=sgl 10.0) -> (x/y=w372:sgl)
              n186 = To Long Integer(number=w373) -> (32bit integer=w375:i32)
              n187 = To Long Integer(number=w372) -> (32bit integer=w376:i32)
              n188 = Subtract(x=w384, y=w375) -> (x-y=w380:i32)
              n189 = Add(x=w382, y=w375) -> (x+y=w378:i32)
              n190 = Add(x=w381, y=w376) -> (x+y=w377:i32)
              n191 = Subtract(x=w383, y=w376) -> (x-y=w379:i32)
            }
            frame True {
              # "****"
              # "if switching states"
              # "Scale / Score"
              # "Main ROI"
              # "Horizontal Scale \n(smaller number = smaller ROI)"
              n192 = case shown="-1" w395 {
                tunnel: w420 -> [w425 w430 w435]
                tunnel: [w424 w426 w431] -> w403
                tunnel: w402 -> [w423 w429 w434]
                tunnel: [w422 w427 w432] -> w401
                frame 0, Default {
                  n193 = Subtract(x=w425, y=w423) -> (x-y=w422:dbl)
                  n194 = Add(x=w423, y=w425) -> (x+y=w424:dbl)
                }
                frame 1 {
                  n195 = Subtract(x=w430, y=5.0) -> (x-y=w427:dbl)
                  n196 = Add(x=w429, y=w430) -> (x+y=w426:dbl)
                }
                frame -1 {
                  n197 = Subtract(x=w435, y=w434) -> (x-y=w432:dbl)
                  n198 = Add(x=5.0 ("y"), y=w435) -> (x+y=w431:dbl)
                }
              }
              n199 = Subtract(x=w421, y=w419) -> (x-y=w418:dbl)
              n200 = Array To Cluster(array=w407) -> (cluster=w417:T13)
              n201 = Unbundle By Name(w417) -> ("Matches (Geometric Matching 1)[0].Position.x"=w411:sgl, "Matches (Geometric Matching 1)[0].Position.y"=w413:sgl, "Matches (Geometric Matching 1)[0].Scale"=w412:sgl)
              n202 = Divide(x=w412, y=w409) -> (x/y=w414:sgl)
              n203 = Multiply(x=w412, y=w408) -> (x*y=w416:sgl)
              n204 = Divide(x=w416, y=sgl 2.0) -> (x/y=w410:sgl)
              n205 = Add(x=w413, y=w414) -> (x+y=w405:sgl)
              n206 = Subtract(x=w413, y=w414) -> (x-y=w406:sgl)
              n207 = Subtract(x=w411, y=w410) -> (x-y=w398:sgl)
              n208 = Add(x=w410, y=w411) -> (x+y=w397:sgl)
              n209 = case shown="False" FALSE {
                tunnel: w404 -> [_ _]
                tunnel: [w438 w447] -> w399
                tunnel: w403 -> [w438 w449]
                tunnel: [w439 w446] -> w400
                tunnel: w401 -> [w439 w448]
                tunnel: w402 -> [_ w445]
                tunnel: [w437 w442] -> _
                tunnel: w398 -> [w437 w443]
                tunnel: [w436 w441] -> _
                tunnel: w397 -> [w436 w444]
                frame False {
                }
                frame True {
                  w440 = sgl 50.0 ("y")
                  # "Double scale cushion\nif changing states"
                  n210 = Add(x=w449, y=w445) -> (x+y=w447:dbl)
                  n211 = Subtract(x=w448, y=w445) -> (x-y=w446:dbl)
                  n212 = Subtract(x=w443, y=w440) -> (x-y=w442:sgl)
                  n213 = Add(x=w440, y=w444) -> (x+y=w441:sgl)
                }
              }
            }
          }
          n214 = Greater?(x=w347, y=w346) -> (0:w348:bool)
          n215 = call "Bound_RO_R_R0I.vi"("Bottom Right - Y"=w351, "Right - X"=w352, "Top Left - Y"=w353, "Top  Left - x"=w354) -> ("ROI Descriptor"=w355:T3)  [unwired: 7 in]
          n216 = Select(t=w347, s=w348, f=w346) -> (s? t:f=w345:dbl)
        }
      }
      "Next Main ROI Descriptor" <- w77
      n217 = Less?(x=w120, y="Absolute\nMinimum Score") -> (x < y?=w124:bool)
      n218 = Less?(x=w90, y="Absolute\nMinimum Scale") -> (x < y?=w93:bool)
      n219 = Greater?(x=w91, y="Absolute\nMaximum Scale") -> (0:w88:bool)
      n220 = Greater?(x=w90, y=w91) -> (0:w94:bool)
      n221 = Less?(x=w91, y=w90) -> (x < y?=w89:bool)
      n222 = Select(t="Absolute\nMinimum Score", s=w124, f=w120) -> (s? t:f=w126:dbl)
      "New Min Score" <- w126
      n223 = Or(x=w93, y=w94) -> (x .or. y?=w95:bool)
      n224 = Or(x=w88, y=w89) -> (x .or. y?=w92:bool)
      n225 = Select(t="Absolute\nMinimum Scale", s=w95, f=w90) -> (s? t:f=w108:dbl)
      "New Low Scale" <- w108
      n226 = Select(t="Absolute\nMaximum Scale", s=w92, f=w91) -> (s? t:f=w109:dbl)
      "New high Scale" <- w109
      n227 = Bundle("index"=w122, "Min Scale"=w108, "Max Scale"=w109) -> (w121:T20)  [unwired: 1 in]
      n228 = Replace Array Subset(array=w119, new element=w121, index=w122) -> (w123:T8[])
      n229 = call "IMAQ Overlay ROI"("ROI Descriptor"=w77, "Image"=w107) -> ("Image Out"=→"Right Image 2":T6)  [unwired: 8 in, 1 out]
      n230 = Bundle By Name(cluster="Current Settings", "Range Settings"=w123, "Minimum Match Score"=w126) -> (→"New Settings":T9)
    }
  }
